vi "PZT_SignalGenerator.vi"(0 "Waveform Type":T1(ring), 1 "Physical Channels":tag="DAQ/ao0", 2 "Offset":dbl=5.0 min=4.0 max=5.0 step=0.0001 format="%0.6p", 3 "Frequency":dbl=1.0 min=0.0 max=100.0 step=0.1 format="%.6f", 4 "PZT_oscillation_stop":bool caption="stop", 5 "Amplitude":dbl=6.0 min=4.0 max=6.0 step=1e-05 format="%0.6p") -> (6 "Waveform Chart":waveform(dbl)(graph)={"t0"=timestamp(6.499999999999999 s since 1904-01-01), "dt"=1e-06, "Y"=array[100000 elements]}, 8 "error out":errorcluster)   [LabVIEW 2017]
doc: "I. Description:\nThis example demonstrates how to continuously output a waveform using an internal sample clock. The automatic regeneration of data has been disabled, so new data has to be provided throughout the duration of the continuous Analog Output operation. This allows the generation of any arbitrary frequency as this VI computes new data for each iteration of the loop, maintaining phase continuity of the signal. The regeneration of data has also been adjusted so that the newest data is output as quickly as possible; thus reducing the lag between the changing of the data and the output of that data.\n\nII. Instructions for Running:\n1. Select the Physical Channel to correspond to where your signal is output on the DAQ device.\n2. Enter the Minimum and Maximum Voltage range.\n3. Specify the desired Sample Clock Rate of the output Waveform. Higher sample clock rates will produce a smoother waveform.\n4. Manually specify the Analog Output buffer size, in number of samples. A larger buffer would help non-regenerative operations avoid errors due to occasional high CPU load. \nNote: \nThe Analog Output buffer has to be at least as big as the amount of data being written to the board per iteration. The recommended buffer size would be at least twice the amount of data being written to the board per iteration.\n5. Enter the Waveform Information. See the documentation of the Basic Function Generator SubVI for information on each parameter.\n\nIII. Block Diagram Steps:\n1. Create an Analog Output Voltage channel.\n2. Configure the task to prohibit the automatic regeneration of data.\n2a. Set the transfer condition to Less than Full. Allows for more rapid updates of Output Buffer.\n3. Call the DAQmx (Sample Clock) VI to set the sample clock rate. Additionally, set the sample mode to Continuous.\n4. Read the actual sample clock rate (eventually coerced depending on the hardware used). \n5. Compute the desired waveform, using the buffer size and the actual update rate. This VI keeps track of the phase of the waveform to ensure that the generated signal is continuous.\n6. Write the waveform to the output buffer. \n7a. Call the Start VI. This is only needed when the loop is executed for the first time.\n7b. Do nothing.\n8. Loop continuously until user presses the Stop button. Every iteration computes and writes a new waveform to the buffer.\n9. Call the Clear Task VI to clear the Task.\n10. Use the popup dialog box to display an error or warning if any.\n\nIV. I/O Connections Overview:\nMake sure your signal output terminal matches the Physical Channel I/O Control. For further connection information, refer to your hardware reference manual."
uses:
  <vilib>/DAQmx/write.llb/DAQmx Write.vi
  <vilib>/DAQmx/create/channels.llb/DAQmx Create Channel (AO-Voltage-Basic).vi
  <vilib>/DAQmx/configure/timing.llb/DAQmx Timing (Sample Clock).vi
  PZT_oscillation.vi
  <vilib>/DAQmx/miscellaneous.llb/DAQmx Fill In Error Info.vi
  <vilib>/measure/NI_MABase.lvlib
  <resource>/objmgr/daqmx.rc
panel:
  in  "Size (Samples)":u32=100000
  out "Actual Sample Clock Rate":dbl=20000.0 format="%.2f"
  in  "Sample Clock Rate":dbl=1000000.0 format="%0.2f"
  in  "Minimum Value":dbl=3.9 min=0.0 max=10.0 step=0.001 format="%0.6f"
  in  "Maximum Value":dbl=6.1 min=0.0 max=10.0 step=0.001 format="%0.6f"
  # "Channel Parameters"
  # "Timing Parameters"
  # "Waveform Information"
  # "Buffer Parameters"
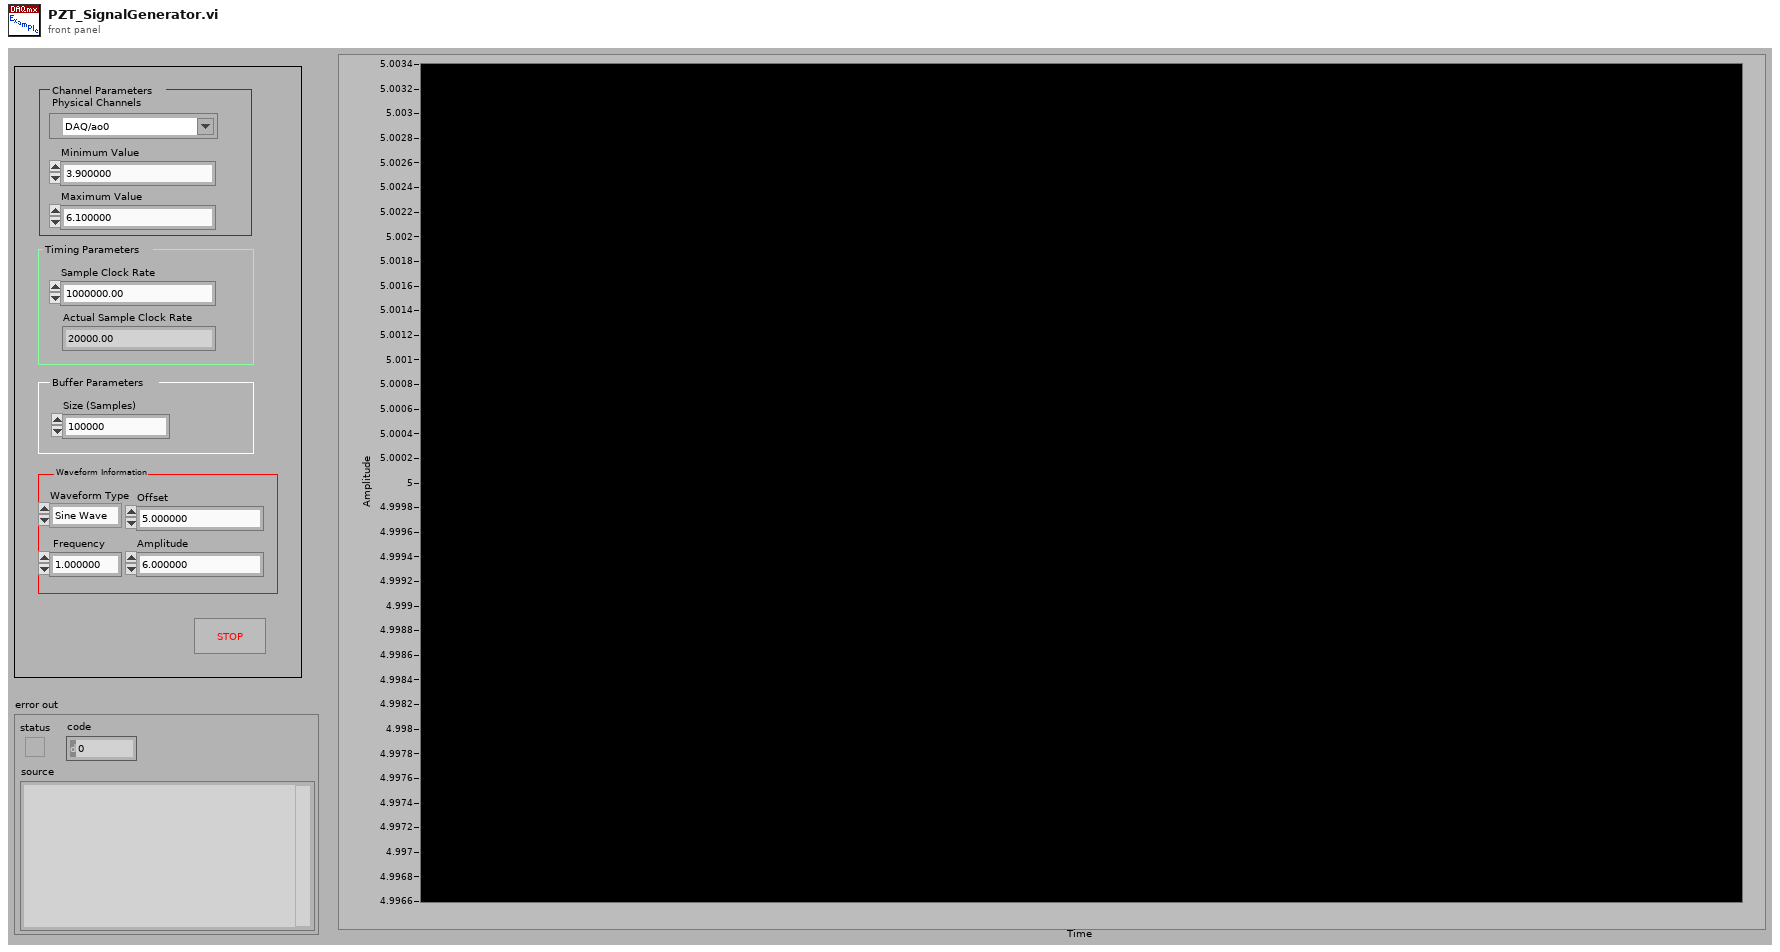
[diagram p1: front panel]
types:
  T1 = enum16{"Sine Wave", "Triangle Wave", "Square Wave", "Sawtooth Wave"}
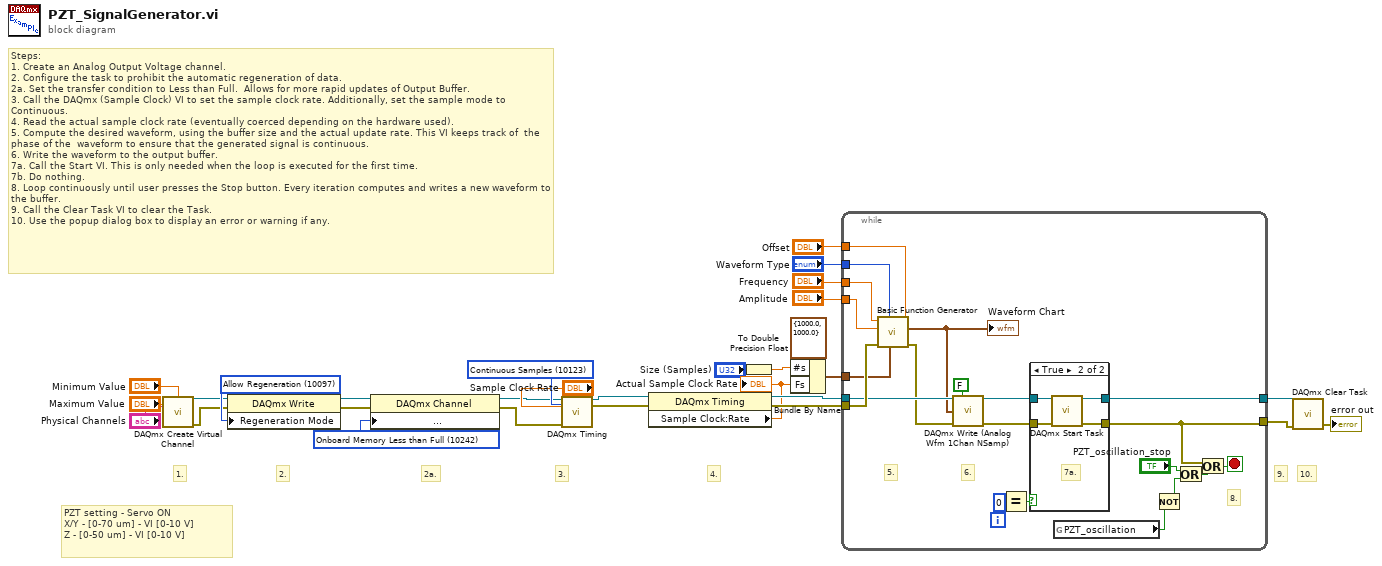
[diagram p0: block diagram]
diagram:
  w10 = 10242 items=["Onboard Memory Empty"=10235, "Onboard Memory Half Full or Less"=10239, "Onboard Memory Less than Full"=10242] ("AO.DataXferReqCond")
  w19 = 10097 items=["Allow Regeneration"=10097, "Do Not Allow Regeneration"=10158] ("RegenMode")
  w28 = 10123 items=["Finite Samples"=10178, "Continuous Samples"=10123] ("sample mode")
  # "PZT setting - Servo ON\nX/Y - [0-70 um] - VI [0-10 V] \nZ - [0-50 um] - VI [0-10 V]"
  # "2a."
  # "4."
  # "3."
  # "Steps:\n1. Create an Analog Output Voltage channel.\n2. Configure the task to prohibit the automatic regeneration of data.\n2a. Set the transfer condition to Less than Full.  Allows for more rapid updates of Output Buffer. \n3. Call the DAQmx (Sample Clock) VI to set the sample clock rate. Additionally, set the sample mode to Continuous.\n4. Read the actual sample clock rate (eventually coerced depending on the hardware used).\n5. Compute the desired waveform, using the buffer size and the actual update rate. This VI keeps track of  the phase of the  waveform to ensure that the generated signal is continuous.\n6. Write the waveform to the output buffer. \n7a. Call the Start VI. This is only needed when the loop is executed for the first time.\n7b. Do nothing.\n8. Loop continuously until user presses the Stop button. Every iteration computes and writes a new waveform to the buffer.\n9. Call the Clear Task VI to clear the Task.\n10. Use the popup dialog box to display an error or warning if any."
  # "10."
  # "9."
  # "2."
  # "1."
  n1 = call-poly <vilib>:"DAQmx Create Virtual Channel.vi"("maximum value"="Maximum Value", "minimum value"="Minimum Value", "physical channels"="Physical Channels") -> ("task out"=w18:refnum<k21>, "error out"=w17:errorcluster)  [unwired: 11 in]
  n2 = property class="DAQmx Write"(reference=w18, error in=w17, "Regeneration Mode"=w19) -> (reference out=w14:refnum<k21>, error out=w11:errorcluster)
  n3 = property class="DAQmx Channel"(reference=w14, error in=w11, "Analog Output:General Properties:Advanced:Data Transfer and Memory:Data Transfer Request Condition"=w10) -> (reference out=w13:refnum<k21>, error out=w12:errorcluster)
  n4 = call-poly <vilib>:"DAQmx Timing.vi"("task/channels in"=w13, "sample mode"=w28, "rate"="Sample Clock Rate", "error in"=w12) -> ("task out"=w22:refnum<k21>, "error out"=w21:errorcluster)  [unwired: 10 in]
  n5 = property class="DAQmx Timing"(reference=w22, error in=w21) -> (reference out=w8:refnum<k21>, error out=w7:errorcluster, "Sample Clock:Rate"=w5:dbl)
  "Actual Sample Clock Rate" <- w5
  n6 = To Double Precision Float(number="Size (Samples)") -> (double precision float=w15:dbl)
  n7 = Bundle By Name(cluster=cluster{"Fs":dbl, "#s":dbl} {"Fs"=1000.0, "#s"=1000.0} ("sampling info"), "#s"=w15, "Fs"=w5) -> (w9:cluster{"Fs":dbl, "#s":dbl})
  n8 = while {
    tunnel: w8 -> [w49]
    tunnel: [w48] -> w24
    tunnel: w7 -> [w51]
    tunnel: [w30] -> w6
    tunnel: w9 -> [w50]
    tunnel: "Offset" -> [w39]
    tunnel: "Waveform Type" -> [w38]
    tunnel: "Frequency" -> [w37]
    tunnel: "Amplitude" -> [w36]
    i -> [w42]
    stop <- w47 stop-if-true
    # "6."
    # "5."
    # "8."
    n9 = call <vilib>:"Basic Function Generator.vi"("offset"=w39, "sampling info"=w50, "signal type"=w38, "error in (no error)"=w51, "amplitude"=w36, "frequency"=w37) -> ("error out"=w46:errorcluster, "signal out"=w31:waveform(dbl))  [unwired: 3 in, 1 out]
    "Waveform Chart" <- w31
    n10 = call-poly <vilib>:"DAQmx Write (Analog Wfm 1Chan NSamp).vi"("task/channels in"=w49, "auto start"=FALSE, "data"=w31, "error in"=w46) -> ("task out"=w45:refnum<k21>, "error out"=w44:errorcluster)  [unwired: 9 in, 1 out]
    n11 = Equal?(x=0, y=w42) -> (x = y?=w40:bool)
    n12 = case shown="True" w40 {
      tunnel: w45 -> [w53 w57]
      tunnel: w44 -> [w52 w56]
      tunnel: [w52 w55] -> w30
      tunnel: [w53 w54] -> w48
      frame False {
        # "7b."
      }
      frame True {
        # "7a."
        n13 = call <vilib>:"DAQmx Start Task.vi"("task/channels in"=w57, "error in"=w56) -> ("task out"=w54:refnum<k21>, "error out"=w55:errorcluster)  [unwired: 12 in]
      }
    }
    n14 = global read "PZT_oscillation.vi" "PZT_oscillation"() -> (w33:bool)
    n15 = Not(x=w33) -> (.not. x?=w32:bool)
    n16 = Or(x="PZT_oscillation_stop", y=w32) -> (x .or. y?=w34:bool)
    n17 = Or(x=w30, y=w34) -> (x .or. y?=w47:bool)
  }
  n18 = call <vilib>:"DAQmx Clear Task.vi"("task in"=w24, "error in"=w6) -> ("error out"=→"error out":errorcluster)  [unwired: 13 in]
